vi "crc_modbus.vi"(5 "input bit":i16[](array[numeric])) -> (1 "crc":i16[](array[numeric]), 2 "output array":i16[](array[numeric]))   [LabVIEW 2014]
panel:
  in  "input string":string="111111110000000010101010"
  out "combined output":string
  out "crc string (hex)":string
  out "crc binary string":string
  out "hex integer string":string
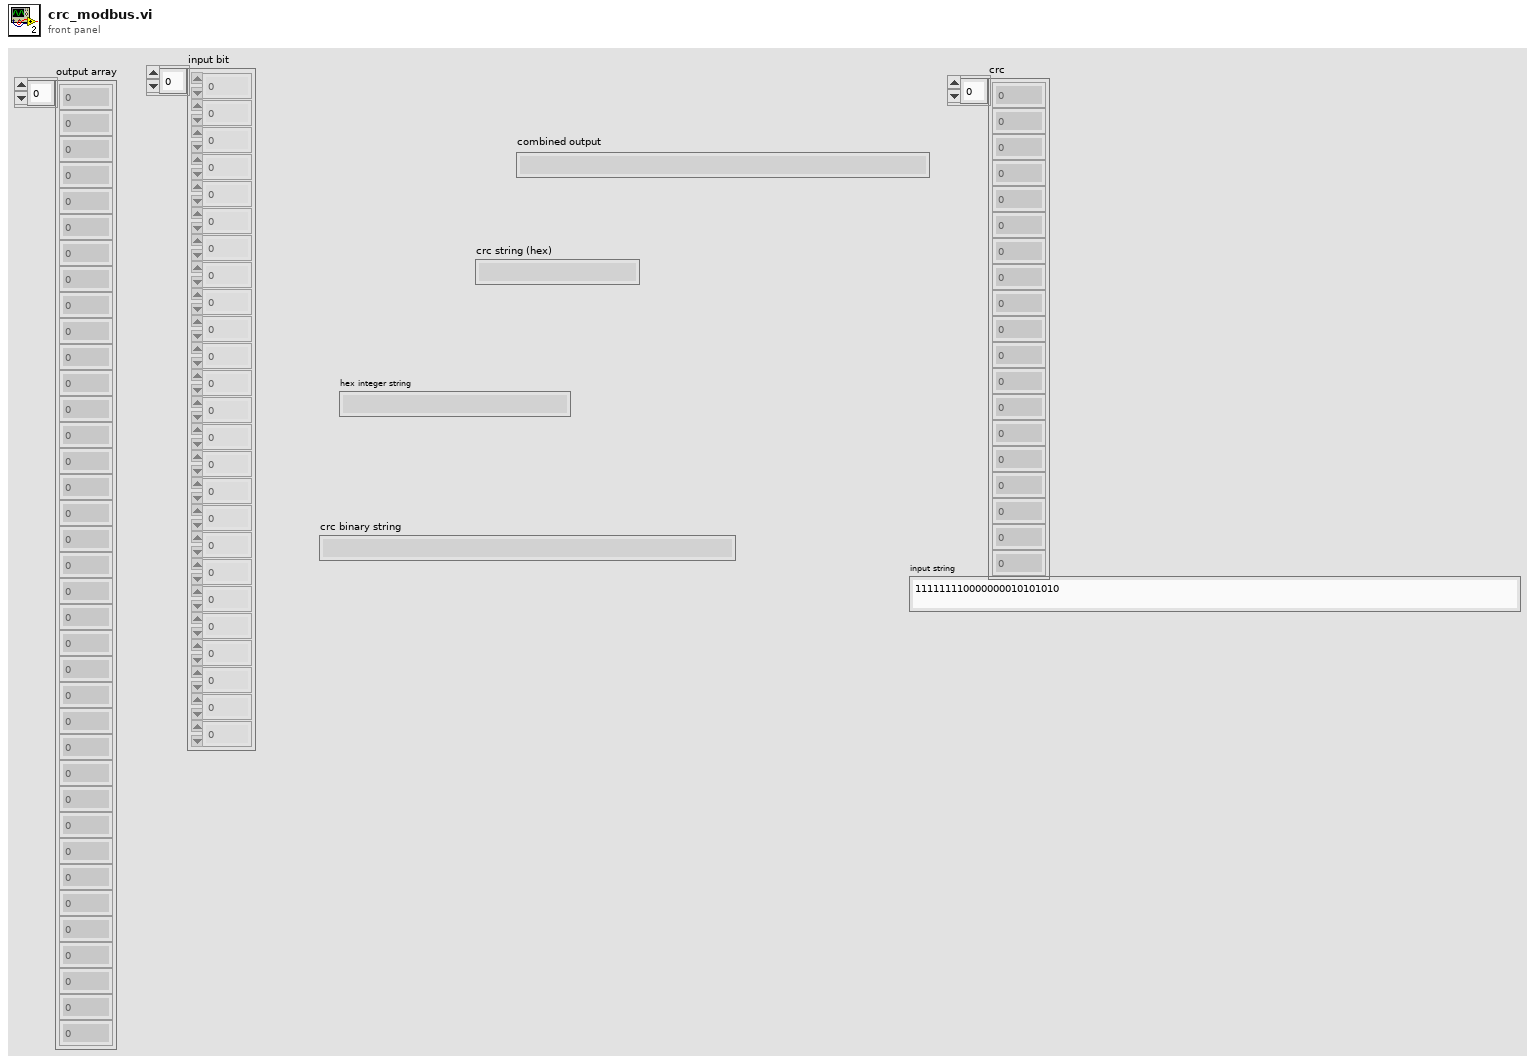
[diagram p1: front panel]
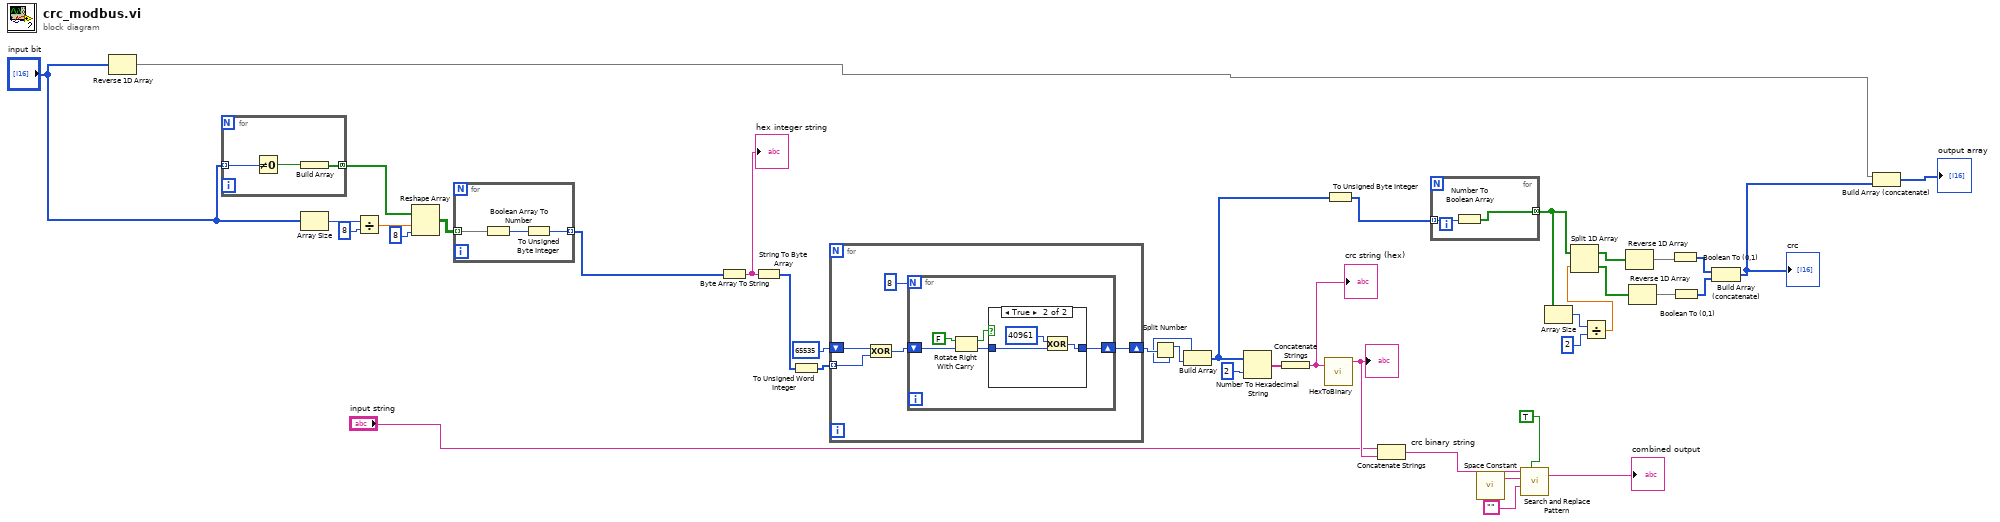
[diagram p0: block diagram]
diagram:
  n1 = Reverse 1D Array(array="input bit") -> (reversed array=w1:i16[])
  n2 = for {
    tunnel: "input bit" -> [w43] mode=indexing
    tunnel: [w41] -> w39 mode=concatenating
    n3 = Not Equal To 0?(x=w43) -> (x != 0?=w42:bool)
    n4 = Build Array(w42) -> (w41:bool[])
  }
  n5 = Array Size(array="input bit") -> (size(s)=w38:i32)
  n6 = Divide(x=w38, y=8) -> (x/y=w36:dbl)
  n7 = Reshape Array(w39, w36, 8) -> (w35:bool[][])
  n8 = for {
    tunnel: w35 -> [w46] mode=indexing
    tunnel: [w44] -> w8 mode=indexing
    n9 = Boolean Array To Number(Boolean array=w46) -> (number=w45:u32)
    n10 = To Unsigned Byte Integer(number=w45) -> (unsigned 8bit integer=w44:u8)
  }
  n11 = Byte Array To String(unsigned byte array=w8) -> (string=w30:string)
  "hex integer string" <- w30
  n12 = String To Byte Array(string=w30) -> (unsigned byte array=w32:u8[])
  n13 = To Unsigned Word Integer(number=w32) -> (unsigned 16bit integer=w31:u16[])
  n14 = for {
    shift-right: [w48] -> w33
    shift-left: u16 65535 -> [w49]
    tunnel: w31 -> [w47] mode=indexing
    n15 = Exclusive Or(1:w47, 2:w49) -> (0:w50:u16)
    n16 = for {
      N: 8 -> [_]
      shift-right: [w55] -> w48
      shift-left: w50 -> [w54]
      n17 = Rotate Right With Carry(2:w54, 3:FALSE ("Übertrag")) -> (0:w56:u16, 1:w53:bool)
      n18 = case shown="True" w53 {
        tunnel: w56 -> [w57 w59]
        tunnel: [w57 w58] -> w55
        frame False {
        }
        frame True {
          n19 = Exclusive Or(1:w59, 2:u16 40961) -> (0:w58:u16)
        }
      }
    }
  }
  n20 = Split Number(x=w33) -> (hi(x)=w6:u8, lo(x)=w5:u8)
  n21 = Build Array(w5, w6) -> (w19:u8[])
  n22 = Number To Hexadecimal String(1:i16 2 ("width (-)"), 2:w19) -> (0:w28:string[])
  n23 = Concatenate Strings(w28) -> (w27:string)
  "crc string (hex)" <- w27
  n24 = call "HexToBinary.vi"("Hex String"=w27) -> ("output string"=w26:string)  [unwired: 1 in, 3 out]
  "crc binary string" <- w26
  n25 = To Unsigned Byte Integer(number=w19) -> (unsigned 8bit integer=w20:u8[])
  n26 = Concatenate Strings("input string", w26) -> (w25:string)
  n27 = for {
    tunnel: w20 -> [w62] mode=indexing
    tunnel: [w61] -> w14 mode=concatenating
    n28 = Number To Boolean Array(number=w62) -> (Boolean array=w61:bool[])
  }
  n29 = call <vilib>:"Space Constant.vi"() -> ("String"=w23:string)
  n30 = call <vilib>:"Search and Replace Pattern.vi"("string"=w25, "regular expression (\"\")"=w23, "replace string (\"\")"="", "replace all? (F)"=TRUE) -> ("result string"=→"combined output":string)  [unwired: 1 in, 1 out]
  n31 = Array Size(array=w14) -> (size(s)=w13:i32)
  n32 = Divide(x=w13, y=2) -> (x/y=w11:dbl)
  n33 = Split 1D Array(array=w14, index=w11) -> (first subarray=w18:bool[], second subarray=w17:bool[])
  n34 = Reverse 1D Array(array=w18) -> (reversed array=w16:bool[])
  n35 = Reverse 1D Array(array=w17) -> (reversed array=w15:bool[])
  n36 = Boolean To (0,1)(Boolean=w16) -> (0, 1=w10:i16[])
  n37 = Boolean To (0,1)(Boolean=w15) -> (0, 1=w9:i16[])
  n38 = Build Array (concatenate)(w10, w9) -> (w4:i16[])
  "crc" <- w4
  n39 = Build Array (concatenate)(w1, w4) -> (→"output array":i16[])
